vi "prueba2ximenacarias.vi"() -> ()   [LabVIEW 2013]
panel:
  out "mayor":dbl
  out "Menor":dbl
  out "Temperatura80":dbl
  out "Promedio":dbl
  out "Velocidad":i32(knob) scale=0.0..220.0
  # "Necesitamos generar 10 velocidades. \nal final de las 10 pruebas presentar :\n-Promedio de las velocidades mayores a 120\n-Velocidad Mayor y menor \n-Cuantas veces la temperatura fue mayor a 80"
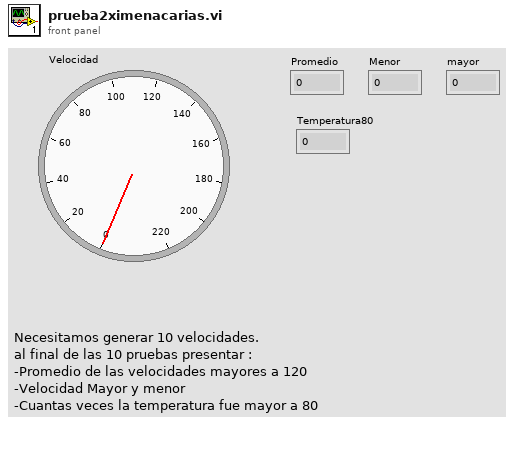
[diagram p1: front panel]
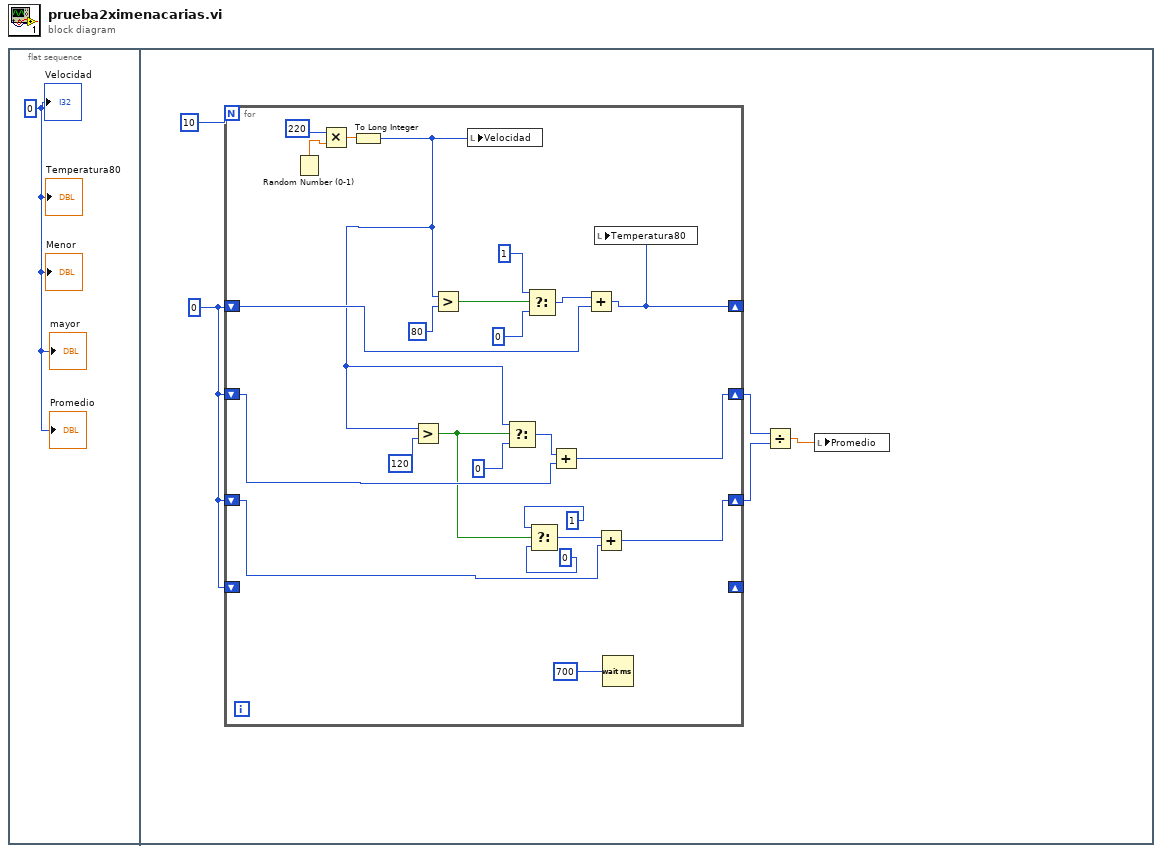
[diagram p0: block diagram]
diagram:
  n1 = flat-sequence {
    frame #0 {
      w1 = 0
      "Velocidad" <- w1
      "Promedio" <- w1
      "Temperatura80" <- w1
      "Menor" <- w1
      "mayor" <- w1
    }
    frame #1 {
      w5 = 0
      n2 = for {
        N: 10 -> [_]
        shift-right: [w20] -> _
        shift-left: w5 -> [w19]
        shift-right: [w7] -> w4
        shift-left: w5 -> [w14]
        shift-right: [w8] -> w3
        shift-left: w5 -> [w9]
        shift-right: _ -> [_]
        shift-left: w5 -> [_]
        n3 = Random Number (0-1)() -> (number: 0 to 1=w28:dbl)
        n4 = Multiply(x=220, y=w28) -> (x*y=w27:dbl)
        n5 = To Long Integer(number=w27) -> (32bit integer=w16:i32)
        n6 = Greater?(x=w16, y=120) -> (0:w13:bool)
        n7 = Greater?(x=w16, y=80) -> (0:w25:bool)
        n8 = local write "Velocidad"(w16) -> ()
        n9 = Select(t=w16, s=w13, f=0) -> (s? t:f=w15:i32)
        n10 = Select(t=1, s=w25, f=0) -> (s? t:f=w22:i32)
        n11 = Select(t=1, s=w13, f=0) -> (s? t:f=w10:i32)
        n12 = Add(x=w15, y=w14) -> (x+y=w7:i32)
        n13 = Add(x=w22, y=w19) -> (x+y=w20:i32)
        n14 = local write "Temperatura80"(w20) -> ()
        n15 = Add(x=w10, y=w9) -> (x+y=w8:i32)
        n16 = Wait (ms)(milliseconds to wait=700) -> ()  [unwired: 1 out]
      }
      n17 = Divide(x=w4, y=w3) -> (x/y=w2:dbl)
      n18 = local write "Promedio"(w2) -> ()
    }
  }
